vi "awgn.vi"() -> ()   [LabVIEW 2020]
uses:
  <vilib>/Platform/TimedLoop/XDataNode/timing_clust.ctl
  <vilib>/Platform/TimedLoop/XDataNode/nitl_modes.ctl
  <vilib>/Platform/TimedLoop/XDataNode/wakeup.ctl
  <vilib>/rvi/FXPMathLib/FxpSinAndCos/subVIs/nifxpmath_SinAndCos_SimConfig.ctl
  <vilib>/rvi/Analysis/measure/FFT/simModelSupport/niFPGA FFT Streaming Sim Properties.ctl
  <vilib>/rvi/Analysis/measure/FFT/simModelSupport/niFPGA FFT Sim Stream Group Properties.ctl
  <vilib>/rvi/Analysis/measure/FFT/simModelSupport/niFPGA FFT Sim Types.ctl
  <vilib>/rvi/Analysis/measure/FFT/simModelSupport/niFpgaFFTSimArithmeticProperties.ctl
  <vilib>/rvi/Analysis/measure/FFT/simModelSupport/niFpgaFFTSimDfxp.ctl
  <vilib>/fxp/LVFixedPointQuantizationPolicyTypeDef.ctl
  <vilib>/rvi/Analysis/measure/FFT/XNode/niFpgaFFTButterflyDelays.ctl
  <vilib>/rvi/Emulation/niFpgaSctlEmulationGetInTimedLoop.vi
  <vilib>/rvi/Emulation/niFpgaEmulationReportErrorSimple.vi
  <vilib>/rvi/Emulation/niFpgaGetClockAttributes.vi
  <vilib>/rvi/Emulation/niFpgaCriticalErrorInLSC.vi
  <vilib>/rvi/interface/RandomDataEmulation/niFpgaRandomDataHandleErrors.vi
  <vilib>/rvi/FXPMathLib/FxpSinAndCos/simVIs/DllFxpSinAndCosTemp_sub.vi
  <vilib>/rvi/Emulation/niFpgaEmulationIsFPGAContextNoSignature.vi
  <vilib>/rvi/errors/niFpgaSetErrorForExecOnDevCompSimple.vi
  <vilib>/rvi/eio/common/nirviEmuReportErrorAndStop.vi
  <vilib>/rvi/DataTransferAndStorage/Container/Common/niFpgaContainerGetUniqueNameForEmu.vi
  <vilib>/rvi/FIFO/Fifo_Resource/nirvififoEmulationSetSize.vi
  <vilib>/rvi/FIFO/Fifo_Resource/nirviFifoEmulationQueueMgr.vi
  <instcachedir>/0/nirviFifoEmulationQueueMgr_E5CAEC123FF24DC58D834DCA3CDAA9B5.lvgen/nirviFifoEmulationQueueMgr_E5CAEC123FF24DC58D834DCA3CDAA9B5_012.vi
  <vilib>/rvi/FIFO/Fifo_Resource/nirvififoEmulationDetermineInputValidOut.vi
  <vilib>/rvi/FIFO/Fifo_Resource/nirvififoEmulationCreateLock.vi
  <vilib>/rvi/Emulation/niFpgaProcessEmulError.vi
  <vilib>/rvi/FIFO/Fifo_Resource/nirvififoEmulationObtainLock.vi
  <vilib>/rvi/FIFO/Fifo_Resource/nirvififoEmulationReleaseLock.vi
  <vilib>/rvi/occurrence/nirviWaitOnOccurrenceBase.vi
  <vilib>/rvi/errors/nirviReportUnexpectedCaseInternalError.vi
  <vilib>/rvi/errors/nirviReportUnexpectedCaseInternalError (U32).vi
  <vilib>/Utility/error.llb/Clear Errors.vi
  <vilib>/rvi/Analysis/measure/FFT/simModelSupport/niFpgaFFTSimModelStreamingCore.vi
  <vilib>/platform/TimedLoop/XDataNode/XDataNode.xnode
  <vilib>/rvi/FXPMathLib/FxpInterpret/XNode/nifxpmath_Interpret.xnode
  <vilib>/rvi/DataTransferAndStorage/Container/XNode/niFpgaContainer.xnode
  <vilib>/rvi/interface/RandomDataEmulation/nirviRandomDataFpgaReadWriteTemplate.vi
  <vilib>/rvi/FXPMathLib/FxpMul/XNode/nifxpmath_Multiplier.xnode
  <vilib>/rvi/FXPMathLib/FxpSinAndCos/XNode/nifxpmath_SinAndCos.xnode
  <vilib>/rvi/FIFO/Fifo_Resource/nirvififoEmulationWrite.vi
  <vilib>/rvi/FIFO/Fifo_Resource/nirvififoEmulationRead.vi
  <vilib>/rvi/Analysis/measure/FFT/XNode/niFpgaFFT.xnode
  <vilib>/Platform/TimedLoop/XDataNode/XDNodeRunTimeDep.lvlib
  <vilib>/rvi/FXPMathLib/sim/FxpSim.dll
panel:
  in  "std":fxp<+,8,8> format="%#_8g"
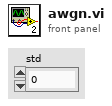
[diagram p1: front panel]
types:
  T1 = typedef "XDNodeRunTimeDep.lvlib/timing_clust.ctl" = cluster{"Expected End [f-1]":u64, "Actual End [f-1]":u64, "Finished Late? [f-1]":bool, "Expected End [i-1]":u64, "Actual End [i-1]":u64, "Finished Late? [i-1]":bool, "Expected Start [i]":u64, "Actual Start [i]":u64, "Expected Start [f]":u64, "Actual Start [f]":u64, "Source Name":string, "Structure Name":string, "Period":i64, "Deadline":i64, "Offset":i64, "Start":i64, "Priority":i32, "Timeout":i32, "Mode":T2, "Wakeup Reason":T3, "Error":errorcluster, "Source Type":string, "Secondary Source Type":string, "Global End Time":u64, "Global Start Time":u64, "Frame Duration":u64, "Iteration Duration":u64, "Assigned CPU":i32, "I/O Scan Engine Mode":u32}
  T2 = typedef "XDNodeRunTimeDep.lvlib/nitl_modes.ctl" = enum32{"No Change", "Process missed periods, maintain original phase", "Discard missed periods, maintain original phase", "Process missed periods, ignore original phase", "Discard missed periods, ignore original phase"}
  T3 = typedef "XDNodeRunTimeDep.lvlib/wakeup.ctl" = enum32{"Normal", "Aborted", "Asynchronous wakeup", "Timing source error", "Timed loop error", "Timeout"}
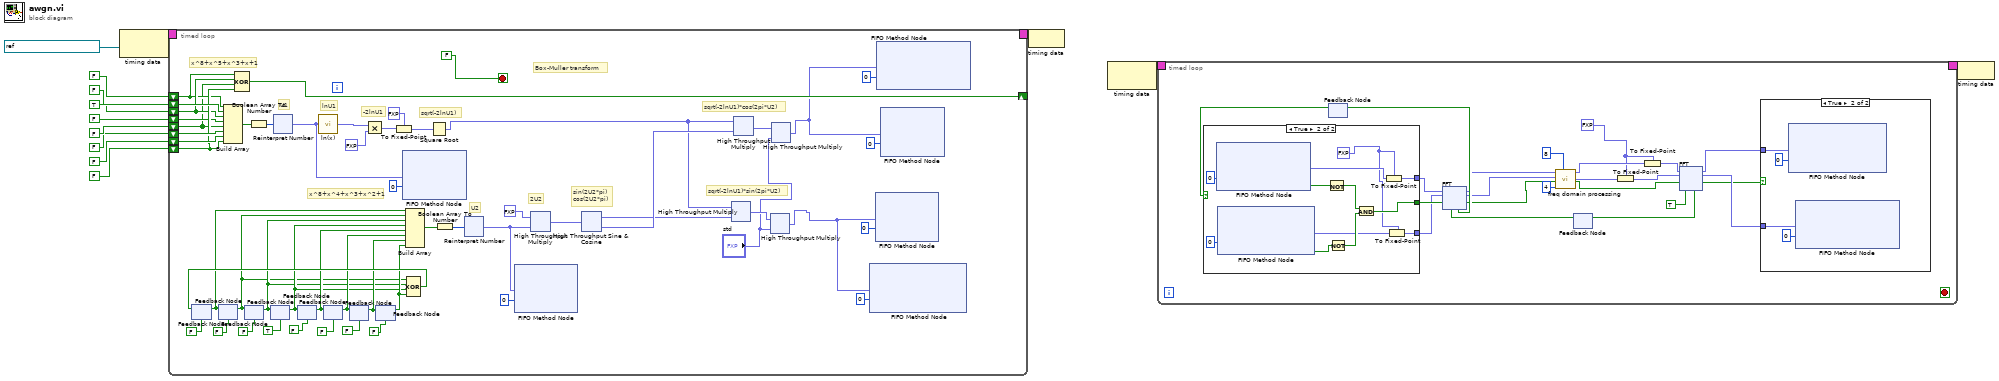
[diagram p0: block diagram]
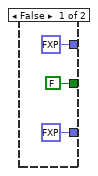
[diagram p3: hidden frame]
diagram:
  n1 = node-c288(refnum<k21> "40 MHz Onboard Clock" ("Source Name")) -> (w13:T1)
  n2 = timed-loop {
    timing: w13 -> [_]
    timing-out: [_] -> w12
    shift-right: [w66] -> _
    shift-left: FALSE -> [w58]
    shift-left: FALSE -> [w65]
    shift-left: TRUE -> [w59]
    shift-left: FALSE -> [w60]
    shift-left: FALSE -> [w57]
    shift-left: FALSE -> [w63]
    shift-left: FALSE -> [w62]
    shift-left: FALSE -> [w61]
    stop <- FALSE stop-if-true
    # "Box-Muller transform"
    # "sqrt(-2lnU1)"
    # "-2lnU1"
    # "lnU1"
    # "sin(2U2*pi)\ncos(2U2*pi)"
    # "sqrt(-2lnU1)*cos(2pi*U2)"
    # "sqrt(-2lnU1)*sin(2pi*U2)"
    # "2U2"
    # "U2"
    # "U1"
    # "x^8+x^4+x^3+x^2+1"
    # "x^8+x^5+x^3+x+1"
    n3 = feedback #1(FALSE) -> (w42:bool)
    n4 = feedback #2(FALSE) -> (w39:bool)
    n5 = feedback-in #2(w42) -> ()
    n6 = Build Array(w58, w65, w59, w60, w57, w63, w62, w61) -> (w64:bool[])
    n7 = Compound Arithmetic op=XOR(w58, w59, w57, w61) -> (w66:bool)
    n8 = feedback #3(FALSE) -> (w40:bool)
    n9 = feedback-in #3(w39) -> ()
    n10 = Boolean Array To Number(Boolean array=w64) -> (number=w56:u8)
    n11 = feedback #4(TRUE) -> (w41:bool)
    n12 = feedback-in #4(w40) -> ()
    n13 = xnode "Reinterpret Number"("x"=w56) -> ("y"=w24:fxp<+,8,0>)
    n14 = feedback #5(FALSE) -> (w43:bool)
    n15 = feedback-in #5(w41) -> ()
    n16 = call "ln(x).vi"("x"=w24) -> ("ln(x)"=w27:fxp<+/-,33,4>)
    n17 = feedback #6(FALSE) -> (w44:bool)
    n18 = feedback-in #6(w43) -> ()
    n19 = feedback #7(FALSE) -> (w45:bool)
    n20 = feedback-in #7(w44) -> ()
    n21 = Multiply(x=w27, y=fxp<+/-,3,2> -2.0) -> (x*y=w31:fxp<+/-,35,5>)
    n22 = feedback #8(FALSE) -> (w46:bool)
    n23 = feedback-in #8(w45) -> ()
    n24 = To Fixed-Point(fixed-point type=fxp<+,18,4> 0.0 ("x*y"), number=w31) -> (fixed-point=w29:fxp<+,18,4>)
    n25 = xnode ("FIFO Method Node")("Element"=w24, "Timeout"=0) -> ()  [unwired: 1 in, 2 out]
    n26 = Build Array(w42, w39, w40, w41, w43, w44, w45, w46) -> (w38:bool[])
    n27 = Compound Arithmetic op=XOR(w39, w40, w41, w46) -> (w55:bool)
    n28 = feedback-in #1(w55) -> ()
    n29 = Square Root(x=w29) -> (sqrt(x)=w28:fxp<+,20,2>)
    n30 = Boolean Array To Number(Boolean array=w38) -> (number=w37:u8)
    n31 = xnode "Reinterpret Number"("x"=w37) -> ("y"=w22:fxp<+,8,0>)
    n32 = xnode ("FIFO Method Node")("Element"=w22, "Timeout"=0) -> ()  [unwired: 1 in, 2 out]
    n33 = xnode "High Throughput Multiply"("x"=fxp<+,2,2> 2.0 ("y"), "y"=w22) -> ("x*y"=w35:fxp<+,10,2>)
    n34 = xnode "High Throughput Sine & Cosine"("x (pi)"=w35) -> ("sin(x)"=w33:fxp<+/-,16,2>, "cos(x)"=w34:fxp<+/-,16,2>)
    n35 = xnode "High Throughput Multiply"("x"=w28, "y"=w33) -> ("x*y"=w15:fxp<+/-,36,4>)
    n36 = xnode "High Throughput Multiply"("x"=w28, "y"=w34) -> ("x*y"=w18:fxp<+/-,36,4>)
    n37 = xnode "High Throughput Multiply"("x"=w15, "y"="std") -> ("x*y"=w16:fxp<+/-,44,12>)
    n38 = xnode "High Throughput Multiply"("x"=w18, "y"="std") -> ("x*y"=w17:fxp<+/-,44,12>)
    n39 = xnode ("FIFO Method Node")("Element"=w16, "Timeout"=0) -> ()  [unwired: 1 in, 2 out]
    n40 = xnode ("FIFO Method Node")("Element"=w16, "Timeout"=0) -> ()  [unwired: 1 in, 2 out]
    n41 = xnode ("FIFO Method Node")("Element"=w17, "Timeout"=0) -> ()  [unwired: 1 in, 2 out]
    n42 = xnode ("FIFO Method Node")("Element"=w17, "Timeout"=0) -> ()  [unwired: 1 in, 2 out]
  }
  n43 = node-c288(w12) -> ()
  n44 = node-c288() -> (w2:T1)  [unwired: 1 in]
  n45 = timed-loop {
    timing: w2 -> [_]
    timing-out: [_] -> w1
    stop <- _ stop-if-true
    w102 = fxp<+/-,24,16> 0.0 ("imaginary data in")
    n46 = feedback #9() -> (w120:bool)  [unwired: 1 in]
    n47 = case shown="True" w120 {
      tunnel: [FALSE w162] -> w121
      tunnel: [fxp<+/-,24,12> 0.0 ("real data in") w160] -> w107
      tunnel: [fxp<+/-,24,12> 0.0 ("real data in") w159] -> w106
      frame False {
      }
      frame True {
        w155 = fxp<+/-,24,12> 0.0 ("real data in")
        n48 = xnode ("FIFO Method Node")("Timeout"=0) -> ("Element"=w156:fxp<+/-,44,12>, "Timed Out?"=w166:bool)  [unwired: 1 in, 1 out]
        n49 = xnode ("FIFO Method Node")("Timeout"=0) -> ("Element"=w161:fxp<+/-,44,12>, "Timed Out?"=w165:bool)  [unwired: 1 in, 1 out]
        n50 = Not(x=w166) -> (.not. x?=w164:bool)
        n51 = Not(x=w165) -> (.not. x?=w163:bool)
        n52 = And(x=w164, y=w163) -> (x .and. y?=w162:bool)
        n53 = To Fixed-Point(fixed-point type=w155, number=w156) -> (fixed-point=w160:fxp<+/-,24,12>)
        n54 = To Fixed-Point(fixed-point type=w155, number=w161) -> (fixed-point=w159:fxp<+/-,24,12>)
      }
    }
    n55 = feedback #10() -> (w118:bool)  [unwired: 1 in]
    n56 = xnode "FFT"("real data in"=w107, "imaginary data in"=w106, "input valid"=w121, "ready for output"=w118) -> ("ready for input"=w119:bool, "real data out"=w105:fxp<+/-,28,16>, "imaginary data out"=w104:fxp<+/-,28,16>, "output valid"=w115:bool)  [unwired: 1 in, 1 out]
    n57 = feedback-in #9(w119) -> ()
    n58 = call "freq domain processing.vi"("fft size"=u16 8, "threshold"=u16 4, "input valid"=w115, "imag data in"=w104, "real data in"=w105) -> ("output valid"=w114:bool, "imag data out"=w113:fxp<+/-,28,16>, "real data out"=w103:fxp<+/-,28,16>)  [unwired: 4 in]
    n59 = To Fixed-Point(fixed-point type=w102, number=w113) -> (fixed-point=w100:fxp<+/-,24,16>)
    n60 = To Fixed-Point(fixed-point type=w102, number=w103) -> (fixed-point=w101:fxp<+/-,24,16>)
    n61 = xnode "FFT"("real data in"=w101, "imaginary data in"=w100, "input valid"=w114, "ready for output"=TRUE) -> ("ready for input"=w109:bool, "real data out"=w111:fxp<+/-,28,17>, "imaginary data out"=w110:fxp<+/-,28,17>, "output valid"=w108:bool)  [unwired: 1 in, 1 out]
    n62 = feedback-in #10(w109) -> ()
    n63 = case shown="True" w108 {
      tunnel: w111 -> [_ w125]
      tunnel: w110 -> [_ w122]
      frame False {
      }
      frame True {
        n64 = xnode ("FIFO Method Node")("Element"=w125, "Timeout"=0) -> ()  [unwired: 1 in, 2 out]
        n65 = xnode ("FIFO Method Node")("Element"=w122, "Timeout"=0) -> ()  [unwired: 1 in, 2 out]
      }
    }
  }
  n66 = node-c288(w1) -> ()
